vi "Get Node by String Address.vi"(8 "error in":errorcluster, 11 "XML Document in":refnum<class "XML Document.lvclass">) -> (0 "error out":errorcluster, 3 "XML Document out":refnum<class "XML Document.lvclass">)   [LabVIEW 2014, in "XML Document.lvclass"]
uses:
  XML Document.lvclass
  Node_class/Node.lvclass
panel:
  out "Found?":bool
  out "Node out":refnum<class "Node.lvclass">
  in  "String Address":string
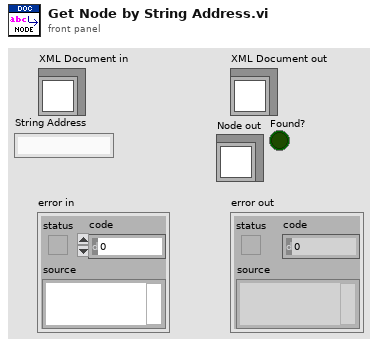
[diagram p1: front panel]
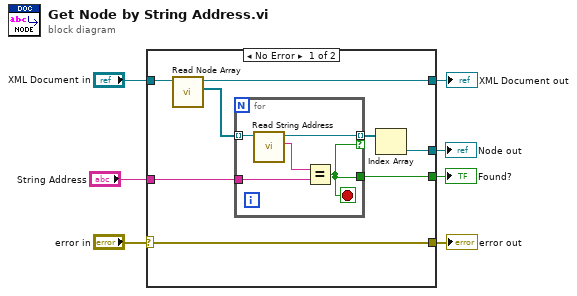
[diagram p0: block diagram]
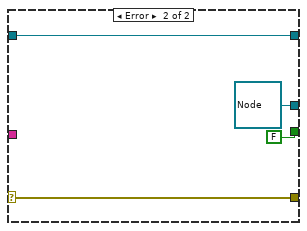
[diagram p2: hidden frame]
diagram:
  n1 = case shown="No Error" "error in" {
    selector: "error in" -> [w14 w24]
    tunnel: [w14 w24] -> w6
    tunnel: [w13 w23] -> w4
    tunnel: "XML Document in" -> [w15 w23]
    tunnel: "String Address" -> [w11 _]
    tunnel: [w9 refnum<class "Node.lvclass"> refnum ("Node out")] -> w2
    tunnel: [w8 FALSE] -> w1
    frame No Error {
      n2 = call-dynamic "Read Node Array.vi"("XML Document in"=w15) -> ("Node Array"=w12:refnum<class "Node.lvclass">[], "XML Document out"=w13:refnum<class "XML Document.lvclass">)  [unwired: 8 in, 1 out]
      n3 = for {
        tunnel: w12 -> [w20] mode=indexing
        tunnel: w11 -> [w18]
        tunnel: [w17] -> w10 mode=indexing if=w16
        tunnel: [w16] -> w8
        stop <- w16 stop-if-true
        n4 = call-dynamic "Read String Address.vi"("Node in"=w20) -> ("String Address"=w19:string, "Node out"=w17:refnum<class "Node.lvclass">)  [unwired: 8 in, 1 out]
        n5 = Equal?(x=w19, y=w18) -> (x = y?=w16:bool)
      }
      n6 = Index Array(array=w10) -> (element=w9:refnum<class "Node.lvclass">)  [unwired: 1 in]
    }
    frame Error {
    }
  }
  "error out" <- w6
  "XML Document out" <- w4
  "Node out" <- w2
  "Found?" <- w1
